vi "Reshape basins.vi"(10 "Array 3":i32[][](array[numeric]), 11 "Array in":bool[][](array[boolean])) -> (2 "Array out":i32[][](array[numeric]), 3 "Boolean":bool)   [LabVIEW 2019, in "Day 9.lvlib"]
uses:
  Day 9.lvlib
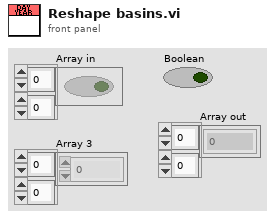
[diagram p1: front panel]
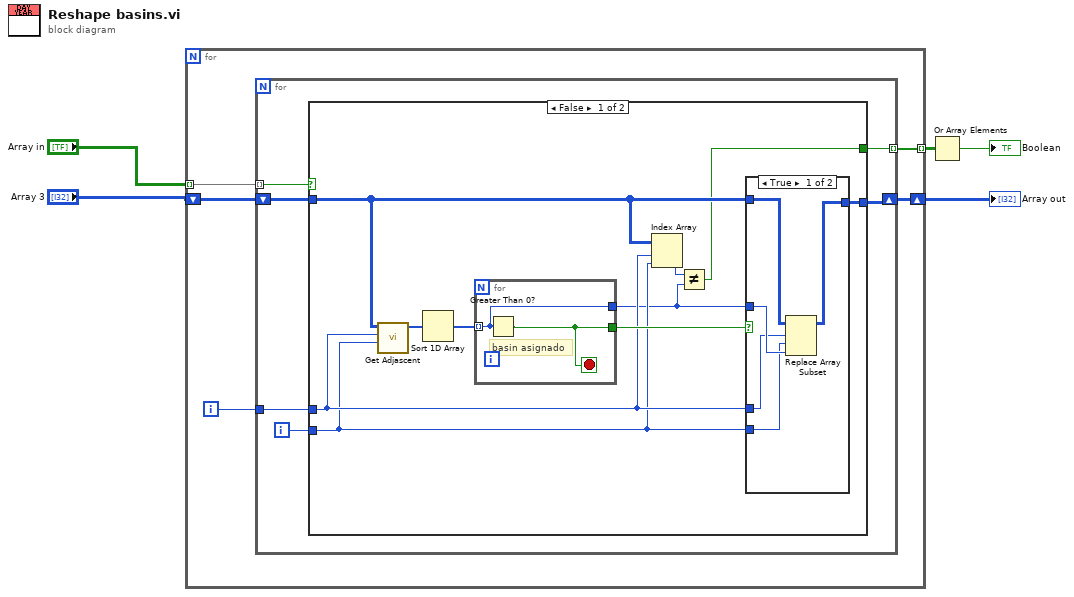
[diagram p0: block diagram]
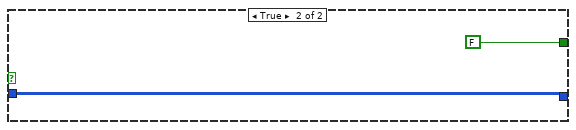
[diagram p3: hidden frame]
diagram:
  n1 = for {
    tunnel: "Array in" -> [w10] mode=indexing
    shift-right: [w7] -> w3
    shift-left: "Array 3" -> [w8]
    tunnel: [w6] -> w4 mode=indexing
    i -> [w9]
    n2 = for {
      tunnel: w10 -> [w16] mode=indexing
      tunnel: w9 -> [w14]
      shift-right: [w12] -> w7
      shift-left: w8 -> [w15]
      tunnel: [w11] -> w6 mode=indexing
      i -> [w13]
      n3 = case shown="False" w16 {
        tunnel: w15 -> [w22 w36]
        tunnel: w14 -> [w21 _]
        tunnel: w13 -> [w20 _]
        tunnel: [w26 w36] -> w12
        tunnel: [w17 FALSE] -> w11
        frame False {
          n4 = call "Get Adjascent.vi"("column"=w20, "row"=w21, "Array in"=w22) -> ("Array out"=w25:i32[])  [unwired: 8 in]
          n5 = Sort 1D Array(array=w25) -> (sorted array=w24:i32[])
          n6 = for {
            tunnel: w24 -> [w28] mode=indexing
            tunnel: [w28] -> w18
            tunnel: [w27] -> w23
            stop <- w27 stop-if-true
            # "basin asignado"
            n7 = Greater Than 0?(x=w28) -> (x > 0?=w27:bool)
          }
          n8 = Index Array(array=w22, index (row)=w21, index (col)=w20) -> (element=w19:i32)
          n9 = Not Equal?(x=w19, y=w18) -> (x != y?=w17:bool)
          n10 = case shown="True" w23 {
            tunnel: w22 -> [w33 w34]
            tunnel: w18 -> [w32 _]
            tunnel: w21 -> [w31 _]
            tunnel: w20 -> [w30 _]
            tunnel: [w29 w34] -> w26
            frame True {
              n11 = Replace Array Subset(array=w33, new element=w32, index (row)=w31, index (col)=w30) -> (w29:i32[][])
            }
            frame False {
            }
          }
        }
        frame True {
        }
      }
    }
  }
  "Array out" <- w3
  n12 = Or Array Elements(Boolean array=w4) -> (logical OR=→"Boolean":bool)
